vi "Security system.vi"() -> ()   [LabVIEW 2024]
uses:
  State of security system.ctl
  Data.ctl
  Active Input.ctl
  <vilib>/Utility/file.llb/Write Delimited Spreadsheet (string).vi
panel:
  out "Zone Status Indicators":T1={"Boolean"=FALSE, "Boolean 2"=FALSE, "Boolean 3"=FALSE, "Boolean 4"=FALSE, "Boolean 5"=TRUE}
  in  "STOP Simulation":bool
  in  "Tamper Switches":bool[](array[boolean])=[FALSE, FALSE, FALSE, FALSE, FALSE]
  in  "Bypass Switches":bool[](array[boolean])=[FALSE, FALSE, FALSE, FALSE, FALSE]
  in  "Alarm Switches":bool[](array[boolean])=[FALSE, FALSE, FALSE, FALSE, FALSE]
  # "Zone"
  # "1"
  # "2"
  # "3"
  # "4"
  # "5"
  # "Green   = Normal\nRed      = Alarm\nOrange = Tamper\nBlue      = Bypass"
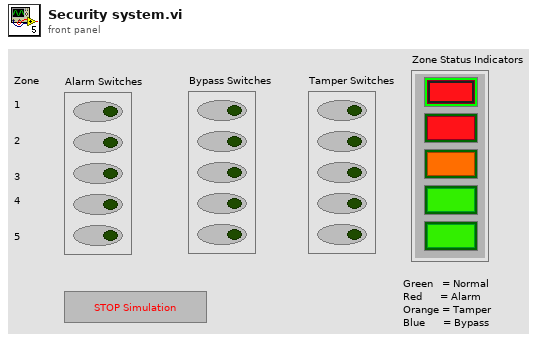
[diagram p1: front panel]
types:
  T1 = cluster{"Boolean":bool, "Boolean 2":bool, "Boolean 3":bool, "Boolean 4":bool, "Boolean 5":bool}
  T2 = typedef "Data.ctl" = cluster{"Active Input for each Zone":T3[], "Alarm Switches":bool[], "Bypass Switches":bool[], "Tamper Switches":bool[], "new file path (Not A Path if cancelled)":path}
  T3 = typedef "Active Input.ctl" = enum16{"Alarm, Bypass & Tamper", "Bypass & Tamper", "Alarm & Tamper", "Alarm & Bypass", "Tamper", "Bypass", "Alarm", "None"}
  T4 = typedef "State of security system.ctl" = enum16{"Initialize", "Wait for triggers", "Alarm", "Bypass", "Tamper", "Exit"}
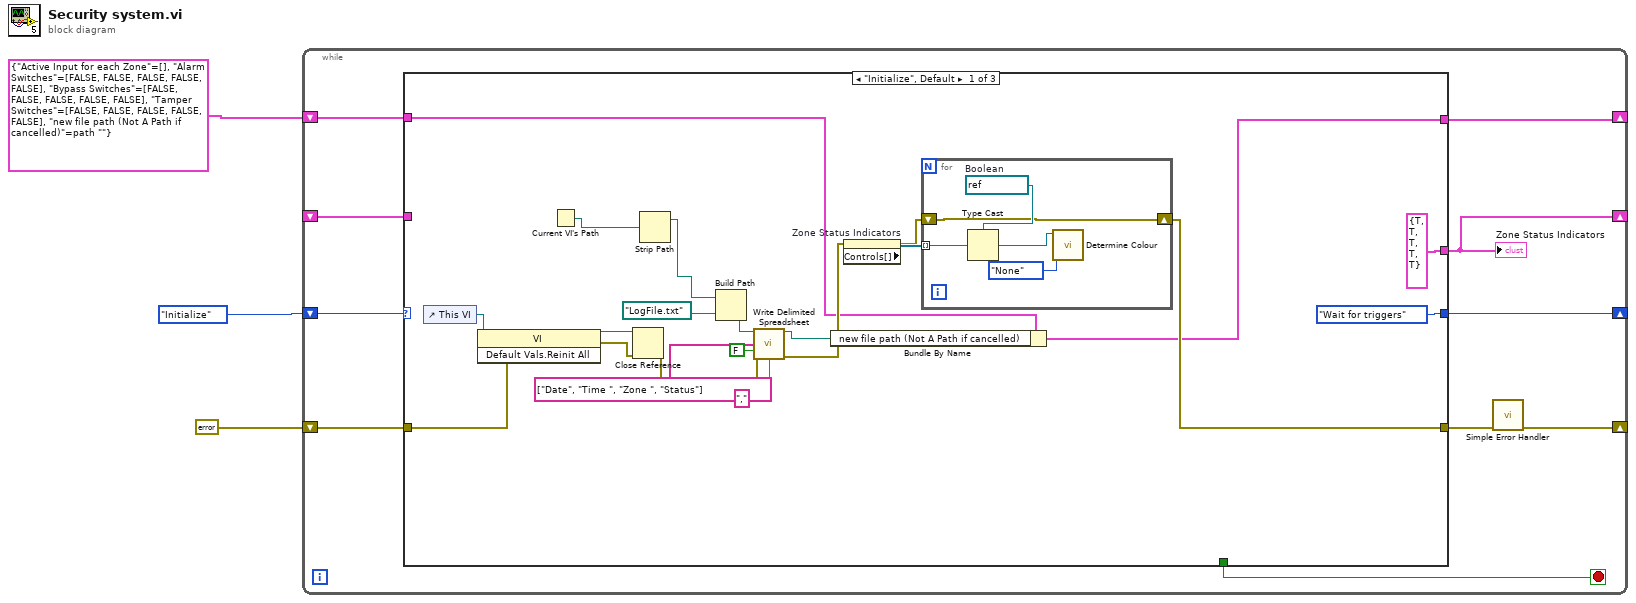
[diagram p0: block diagram]
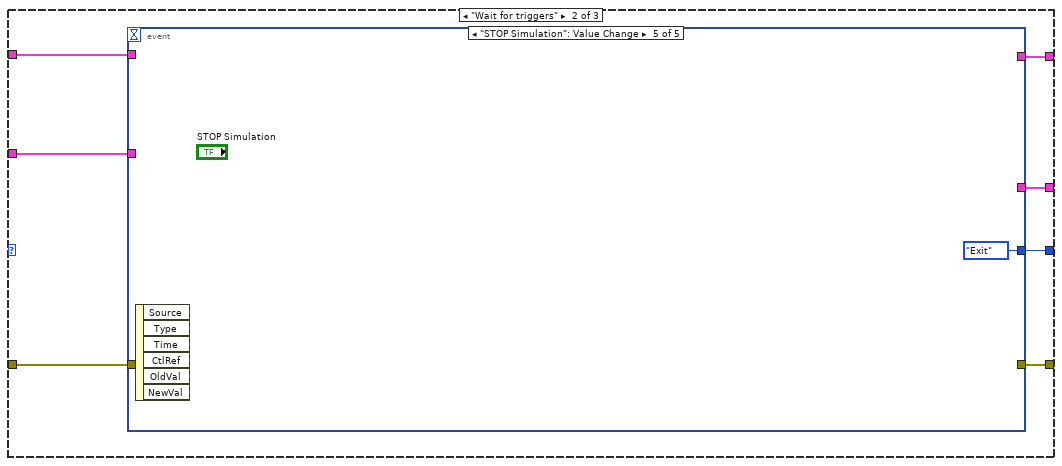
[diagram p2: hidden frame]
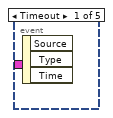
[diagram p3: hidden frame]
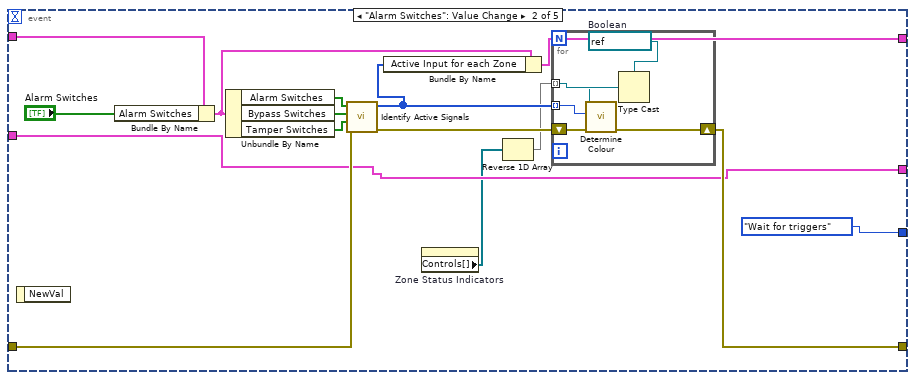
[diagram p4: hidden frame]
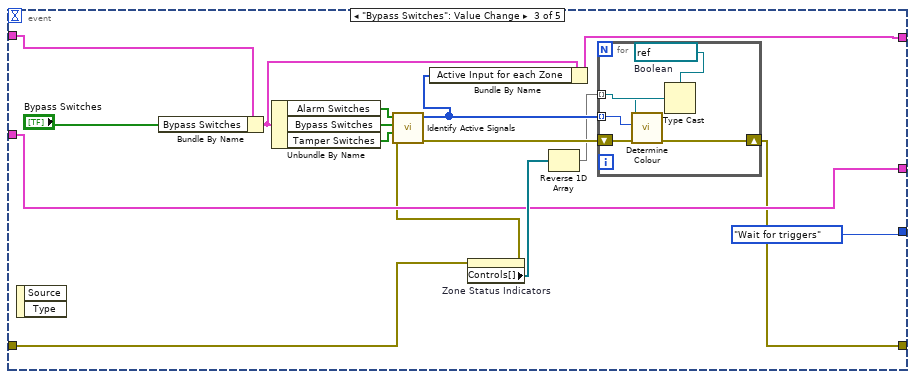
[diagram p5: hidden frame]
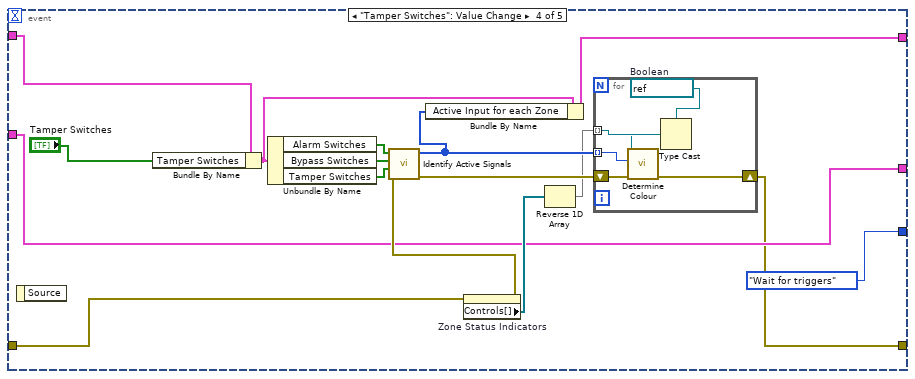
[diagram p6: hidden frame]
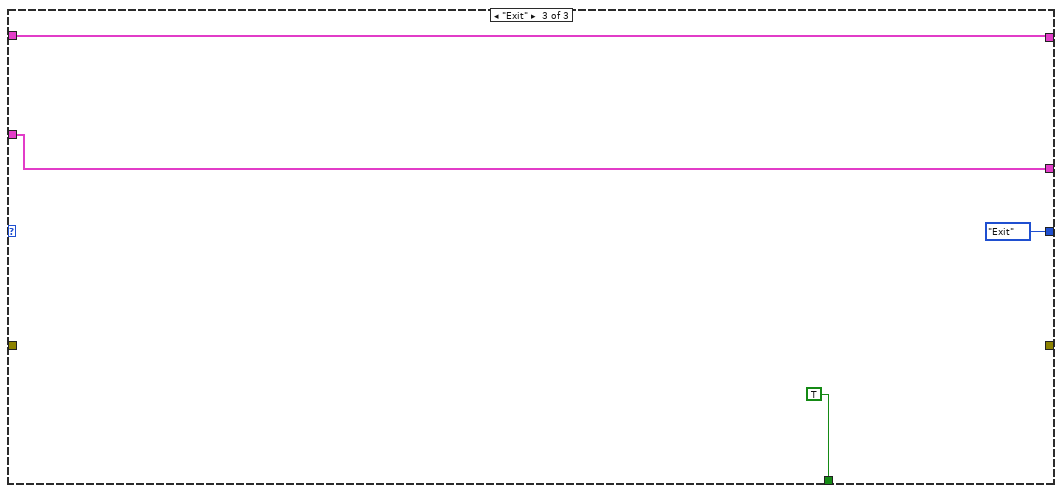
[diagram p7: hidden frame]
diagram:
  n1 = while {
    shift-right: [w12] -> _
    shift-left: State_of_security_system."Initialize" -> [w13]
    shift-right: [w9] -> _
    shift-left: errorcluster {"status"=FALSE, "code"=0, "source"=""} ("error constant") -> [w11]
    shift-right: [w7] -> _
    shift-left: T2 {"Active Input for each Zone"=[], "Alarm Switches"=[FALSE, FALSE, FALSE, FALSE, FALSE], "Bypass Switches"=[FALSE, FALSE, FALSE, FALSE, FALSE], "Tamper Switches"=[FALSE, FALSE, FALSE, FALSE, FALSE], "new file path (Not A Path if cancelled)"=path ""} ("Data") -> [w8]
    shift-right: [w6] -> _
    shift-left: _ -> [w5]
    stop <- w4 stop-if-true
    n2 = case shown="\"Initialize\", Default" w13 {
      tunnel: [T1 {"Boolean"=TRUE, "Boolean 2"=TRUE, "Boolean 3"=TRUE, "Boolean 4"=TRUE, "Boolean 5"=TRUE} ("Zone Status Indicators") w43 w115] -> w6
      tunnel: [State_of_security_system."Wait for triggers" w40 State_of_security_system."Exit"] -> w12
      tunnel: w11 -> [w32 w46 _]
      tunnel: [w20 w42 _] -> w10
      tunnel: w8 -> [w16 w45 w114]
      tunnel: [w14 w41 w114] -> w7
      tunnel: w5 -> [_ w44 w115]
      tunnel: [_ _ TRUE] -> w4
      frame "Initialize", Default {
        n3 = control-ref of="This VI"() -> (w33:refnum<vi>)
        n4 = invoke class="VI" method="Default Vals.Reinit All"(reference=w33, error in=w32) -> (reference out=w31:refnum<vi>, error out=w30:errorcluster)  [unwired: 1 in, 1 out]
        n5 = Current VI's Path() -> (path=w18:path)
        n6 = Close Reference(reference=w31, error in (no error)=w30) -> (error out=w27:errorcluster)
        n7 = Strip Path(path=w18) -> (stripped path=w17:path)  [unwired: 1 out]
        n8 = Build Path(base path=w17, name or relative path=path "LogFile.txt") -> (appended path=w23:path)
        n9 = call-poly <vilib>:"Write Delimited Spreadsheet.vi"("file path (dialog if empty)"=w23, "1D data"=string[] ["Date", "Time ", "Zone ", "Status"], "append to file? (new file:F)"=FALSE, "error in (no error)"=w27, "delimiter (\\t)"="," ("delimiter (\\t)")) -> ("new file path (Not A Path if cancelled)"=w15:path, "error out"=w22:errorcluster)  [unwired: 9 in]
        n10 = Bundle By Name(cluster=w16, "new file path (Not A Path if cancelled)"=w15) -> (w14:T2)
        n11 = property on="Zone Status Indicators" class="Clust (strict)"(error in=w22) -> (error out=w21:errorcluster, "Controls[]"=w29:refnum<vi>[])  [unwired: 1 in, 1 out]
        n12 = for {
          tunnel: w29 -> [w39] mode=indexing
          shift-right: [w35] -> w20
          shift-left: w21 -> [w35]
          w38 = refnum<vi> refnum  # Boolean
          n13 = Type Cast(type=w38, x=w39) -> (*(type *) &x=w37:refnum<vi>)
          n14 = call "Determine Colour.vi"("Active Input"=Active_Input."None", "*(type *) &x"=w37) -> ()  [unwired: 9 in, 1 out]
        }
      }
      frame "Wait for triggers" {
        n15 = event shown="[4] \"STOP Simulation\": Value Change" {
          selector: _ -> [_ _ _ _ _]
          dyn-events: _ -> [_ _ _ _ _]
          timeout: _ -> [_ _ _ _ _]
          tunnel: w46 -> [_ w56 w72 w94 _]
          tunnel: w45 -> [_ w60 w74 w95 _]
          tunnel: w44 -> [_ w49 w73 w93 _]
          tunnel: [_ w49 w73 w93 _] -> w43
          tunnel: [_ w54 w69 w91 _] -> w42
          tunnel: [_ w51 w71 w92 _] -> w41
          tunnel: [_ State_of_security_system."Wait for triggers" State_of_security_system."Wait for triggers" State_of_security_system."Wait for triggers" State_of_security_system."Exit"] -> w40
          event Timeout {
            n16 = event-data() -> ()  [unwired: 1 in, 3 out]
          }
          event "Alarm Switches": Value Change {
            n17 = event-data() -> ()  [unwired: 1 in, 1 out]
            n18 = Bundle By Name(cluster=w60, "Alarm Switches"="Alarm Switches") -> (w53:T2)
            n19 = Unbundle By Name(w53) -> ("Alarm Switches"=w59:bool[], "Bypass Switches"=w58:bool[], "Tamper Switches"=w57:bool[])
            n20 = call "Identify Active Signals.vi"("Error In"=w56, "Tamper Switches"=w57, "Bypass Switches"=w58, "Alarm Switches"=w59) -> ("Error Out"=w55:errorcluster, "Active Input for each Zone"=w52:T3[])  [unwired: 6 in]
            n21 = Bundle By Name(cluster=w53, "Active Input for each Zone"=w52) -> (w51:T2)
            n22 = property on="Zone Status Indicators" class="Clust (strict)"() -> ("Controls[]"=w48:refnum<vi>[])  [unwired: 2 in, 2 out]
            n23 = Reverse 1D Array(array=w48) -> (reversed array=w47:refnum<vi>[])
            n24 = for {
              tunnel: w52 -> [w67] mode=indexing
              shift-right: [w65] -> w54
              shift-left: w55 -> [w66]
              tunnel: w47 -> [w63] mode=indexing
              w64 = refnum<vi> refnum  # Boolean
              n25 = Type Cast(type=w64, x=w63) -> (*(type *) &x=w62:refnum<vi>)
              n26 = call "Determine Colour.vi"("Error In"=w66, "Active Input"=w67, "*(type *) &x"=w62) -> ("Error Out"=w65:errorcluster)  [unwired: 8 in]
            }
          }
          event "Bypass Switches": Value Change {
            n27 = event-data() -> ()  [unwired: 1 in, 2 out]
            n28 = Bundle By Name(cluster=w74, "Bypass Switches"="Bypass Switches") -> (w79:T2)
            n29 = Unbundle By Name(w79) -> ("Alarm Switches"=w83:bool[], "Bypass Switches"=w82:bool[], "Tamper Switches"=w81:bool[])
            n30 = property on="Zone Status Indicators" class="Clust (strict)"(error in=w72) -> (error out=w70:errorcluster, "Controls[]"=w77:refnum<vi>[])  [unwired: 1 in, 1 out]
            n31 = call "Identify Active Signals.vi"("Error In"=w70, "Tamper Switches"=w81, "Bypass Switches"=w82, "Alarm Switches"=w83) -> ("Error Out"=w80:errorcluster, "Active Input for each Zone"=w78:T3[])  [unwired: 6 in]
            n32 = Bundle By Name(cluster=w79, "Active Input for each Zone"=w78) -> (w71:T2)
            n33 = Reverse 1D Array(array=w77) -> (reversed array=w76:refnum<vi>[])
            n34 = for {
              tunnel: w78 -> [w89] mode=indexing
              shift-right: [w87] -> w69
              shift-left: w80 -> [w88]
              tunnel: w76 -> [w85] mode=indexing
              w86 = refnum<vi> refnum  # Boolean
              n35 = Type Cast(type=w86, x=w85) -> (*(type *) &x=w84:refnum<vi>)
              n36 = call "Determine Colour.vi"("Error In"=w88, "Active Input"=w89, "*(type *) &x"=w84) -> ("Error Out"=w87:errorcluster)  [unwired: 8 in]
            }
          }
          event "Tamper Switches": Value Change {
            n37 = event-data() -> ()  [unwired: 1 in, 1 out]
            n38 = Bundle By Name(cluster=w95, "Tamper Switches"="Tamper Switches") -> (w101:T2)
            n39 = Unbundle By Name(w101) -> ("Alarm Switches"=w105:bool[], "Bypass Switches"=w104:bool[], "Tamper Switches"=w103:bool[])
            n40 = property on="Zone Status Indicators" class="Clust (strict)"(error in=w94) -> (error out=w97:errorcluster, "Controls[]"=w99:refnum<vi>[])  [unwired: 1 in, 1 out]
            n41 = call "Identify Active Signals.vi"("Error In"=w97, "Tamper Switches"=w103, "Bypass Switches"=w104, "Alarm Switches"=w105) -> ("Error Out"=w102:errorcluster, "Active Input for each Zone"=w100:T3[])  [unwired: 6 in]
            n42 = Bundle By Name(cluster=w101, "Active Input for each Zone"=w100) -> (w92:T2)
            n43 = Reverse 1D Array(array=w99) -> (reversed array=w98:refnum<vi>[])
            n44 = for {
              tunnel: w100 -> [w111] mode=indexing
              shift-right: [w109] -> w91
              shift-left: w102 -> [w110]
              tunnel: w98 -> [w107] mode=indexing
              w108 = refnum<vi> refnum  # Boolean
              n45 = Type Cast(type=w108, x=w107) -> (*(type *) &x=w106:refnum<vi>)
              n46 = call "Determine Colour.vi"("Error In"=w110, "Active Input"=w111, "*(type *) &x"=w106) -> ("Error Out"=w109:errorcluster)  [unwired: 8 in]
            }
          }
          event "STOP Simulation": Value Change {
            n47 = event-data() -> ()  [unwired: 1 in, 6 out]
          }
        }
      }
      frame "Exit" {
      }
    }
    "Zone Status Indicators" <- w6
    n48 = call <vilib>:"Simple Error Handler.vi"("error in (no error)"=w10) -> ("error out"=w9:errorcluster)  [unwired: 4 in, 4 out]
  }
